vi "Polynom_Stricherl.vi"(6 "Sprachliste":string[][](array[string]), 8 "error in (no error)":errorcluster caption="Fehler (Eingang, kein Fehler)", 9 "Vorschlag Ordnung":i32, 10 "Polynom-Ordnung":T1, 11 "Polynomkoeff.":T2) -> (0 "error out":errorcluster caption="Fehler (Ausgang)", 1 "Vorschlag Ordnung String":string, 2 "Ordnung festgelegt String":string, 3 "Polynom String Array":string[](array[string]))   [LabVIEW 2020, in "Linearisierung v2.lvlib" / "Protokoll.lvlib"]
uses:
  Protokoll.lvlib
  Auswahl Polynom Ordnung.ctl
  Linearisierung v2.lvlib
  Sprachverwaltung/Sprachverwaltung.lvlib
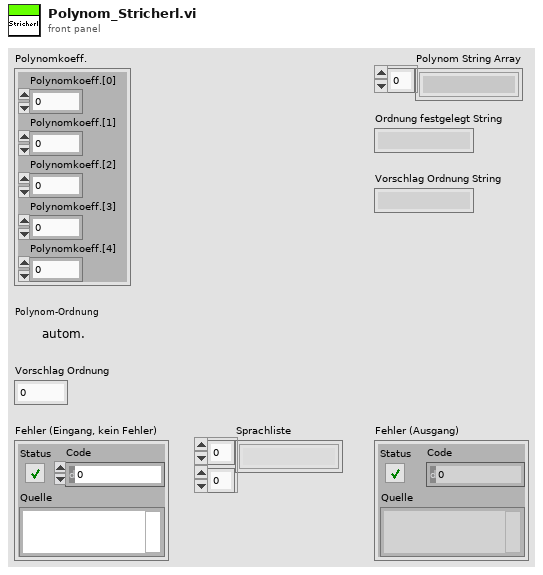
[diagram p1: front panel]
types:
  T1 = typedef "Linearisierung v2.lvlib/Auswahl Polynom Ordnung.ctl" = enum16{"autom.", "raw", "actual", "1", "2", "3", "4"}
  T2 = cluster{"Polynomkoeff.[0]":dbl, "Polynomkoeff.[1]":dbl, "Polynomkoeff.[2]":dbl, "Polynomkoeff.[3]":dbl, "Polynomkoeff.[4]":dbl}
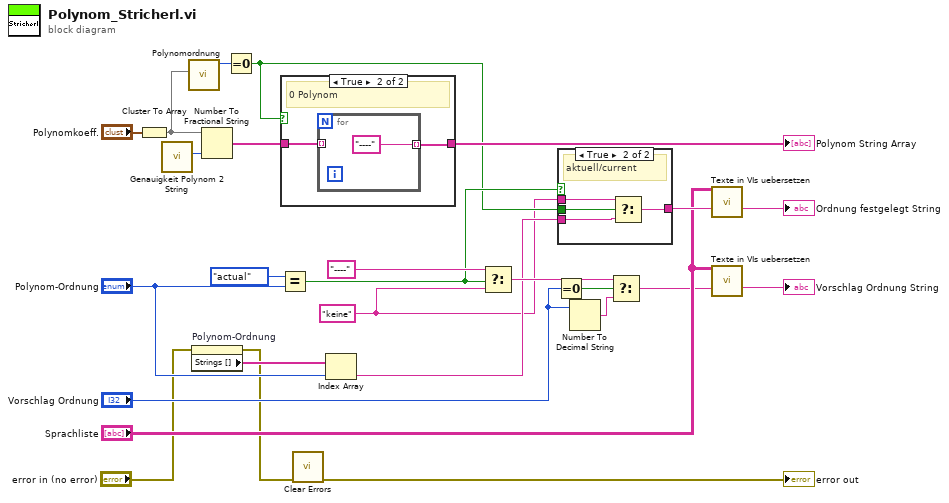
[diagram p0: block diagram]
diagram:
  w10 = "keine" ("String zum Übersetzen")
  n1 = Cluster To Array(cluster="Polynomkoeff.") -> (array=w22:dbl[])
  n2 = call "Genauigkeit Polynom 2 String.vi"() -> ("Genauigkeit für Anzeige"=w25:i16)  [unwired: 9 in, 2 out]
  n3 = call "Polynomordnung.vi"("LIN Polynom"=w22) -> ("Polynomordnung"=w21:i32)  [unwired: 9 in, 1 out]
  n4 = property on="Polynom-Ordnung" class="Enum (strikt)"(error in="error in (no error)") -> (error out=w2:errorcluster, "Strings []"=w20:string[])  [unwired: 1 in, 1 out]
  n5 = Number To Fractional String(number=w22, precision (6)=w25) -> (F-format string=w24:string[])  [unwired: 2 in]
  n6 = Equal To 0?(x=w21) -> (x = 0?=w11:bool)
  n7 = Equal?(x=Auswahl_Polynom_Ordnung."actual", y="Polynom-Ordnung") -> (x = y?=w13:bool)
  n8 = case shown="True" w11 {
    tunnel: w24 -> [w27 w29]
    tunnel: [w27 w28] -> w23
    frame False {
    }
    frame True {
      # "0 Polynom"
      n9 = for {
        tunnel: w29 -> [_] mode=indexing
        tunnel: ["----"] -> w28 mode=indexing
      }
    }
  }
  "Polynom String Array" <- w23
  n10 = call <vilib>:"Clear Errors.vi"("error in (no error)"=w2) -> ("error out"=→"error out":errorcluster)  [unwired: 5 in, 1 out]
  n11 = Index Array(array=w20, index="Polynom-Ordnung") -> (element=w12:string)
  n12 = Select(t="----", s=w13, f=w10) -> (s? t:f=w14:string)
  n13 = Equal To 0?(x="Vorschlag Ordnung") -> (x = 0?=w16:bool)
  n14 = case shown="True" w13 {
    tunnel: w12 -> [w31 w34]
    tunnel: [w31 w33] -> w8
    tunnel: w11 -> [_ w35]
    tunnel: w10 -> [_ w32]
    frame False {
    }
    frame True {
      # "aktuell/current"
      n15 = Select(t=w32, s=w35, f=w34) -> (s? t:f=w33:string)
    }
  }
  n16 = Number To Decimal String(number="Vorschlag Ordnung") -> (decimal integer string=w15:string)  [unwired: 1 in]
  n17 = Select(t=w14, s=w16, f=w15) -> (s? t:f=w5:string)
  n18 = call "Texte in VIs uebersetzen.vi"("Sprachliste"="Sprachliste", "String zum Übersetzen"=w8) -> ("String zum Übersetzen"=→"Ordnung festgelegt String":string)  [unwired: 9 in, 4 out]
  n19 = call "Texte in VIs uebersetzen.vi"("Sprachliste"="Sprachliste", "String zum Übersetzen"=w5) -> ("String zum Übersetzen"=→"Vorschlag Ordnung String":string)  [unwired: 9 in, 4 out]
